vi "main.vi"() -> ()   [LabVIEW 2026]
uses:
  controls/message.ctl
  controls/data.ctl
  controls/channels.ctl
  controls/init cluster.ctl
  <instrlib>/Agilent 2000 3000 X-Series/Agilent 2000 3000 X-Series.lvlib
panel:
  out "times array":timestamp[](array[timestamp])
  in  "File Path":path
  out "results array 2":cluster{"V":dbl, "dV":dbl, "Q":dbl, "dQ":dbl}[](array[cluster])
  out "results array 1":cluster{"V":dbl, "dV":dbl, "Q":dbl, "dQ":dbl}[](array[cluster])
  in  "stop":bool
  out "dQ2":dbl
  out "Q2":dbl
  out "dV2":dbl
  out "V2":dbl
  out "dQ1":dbl
  out "Q1":dbl
  out "dV1":dbl
  out "V1":dbl
  in  "measure way":enum16{"single", "continuous"}(ring)
  in  "Testing":bool
  in  "Scope name":refnum<visa-resource-name>
  out "Initialized":bool
  in  "save":bool
  in  "Stop":bool
  in  "begin":bool
  out "Status":string
  in  "Tab Control":enum32{"Measurement Mode", "Tuning Mode"}(tab)
  out "output 2":waveform(dbl)(graph)
  out "output 1":waveform(dbl)(graph)
  in  "output 2 channel":T1(ring)
  in  "output 1 channel":T2(ring)
  out "output view":waveform(dbl)(graph)
  out "signal and timing":waveform(dbl)[](graph)
  # "CONTROLS"
  # "RESULTS - BCM 1"
  # "RESULTS - BCM 2"
  # "OPERATIONS"
  # "±"
  # "±"
  # "±"
  # "±"
  # "Save to location:"
  # "OUTPUT - BCM 1"
  # "OUTPUT - BCM 2"
  # "SIGNAL AND TIMING"
  # "OUTPUT"
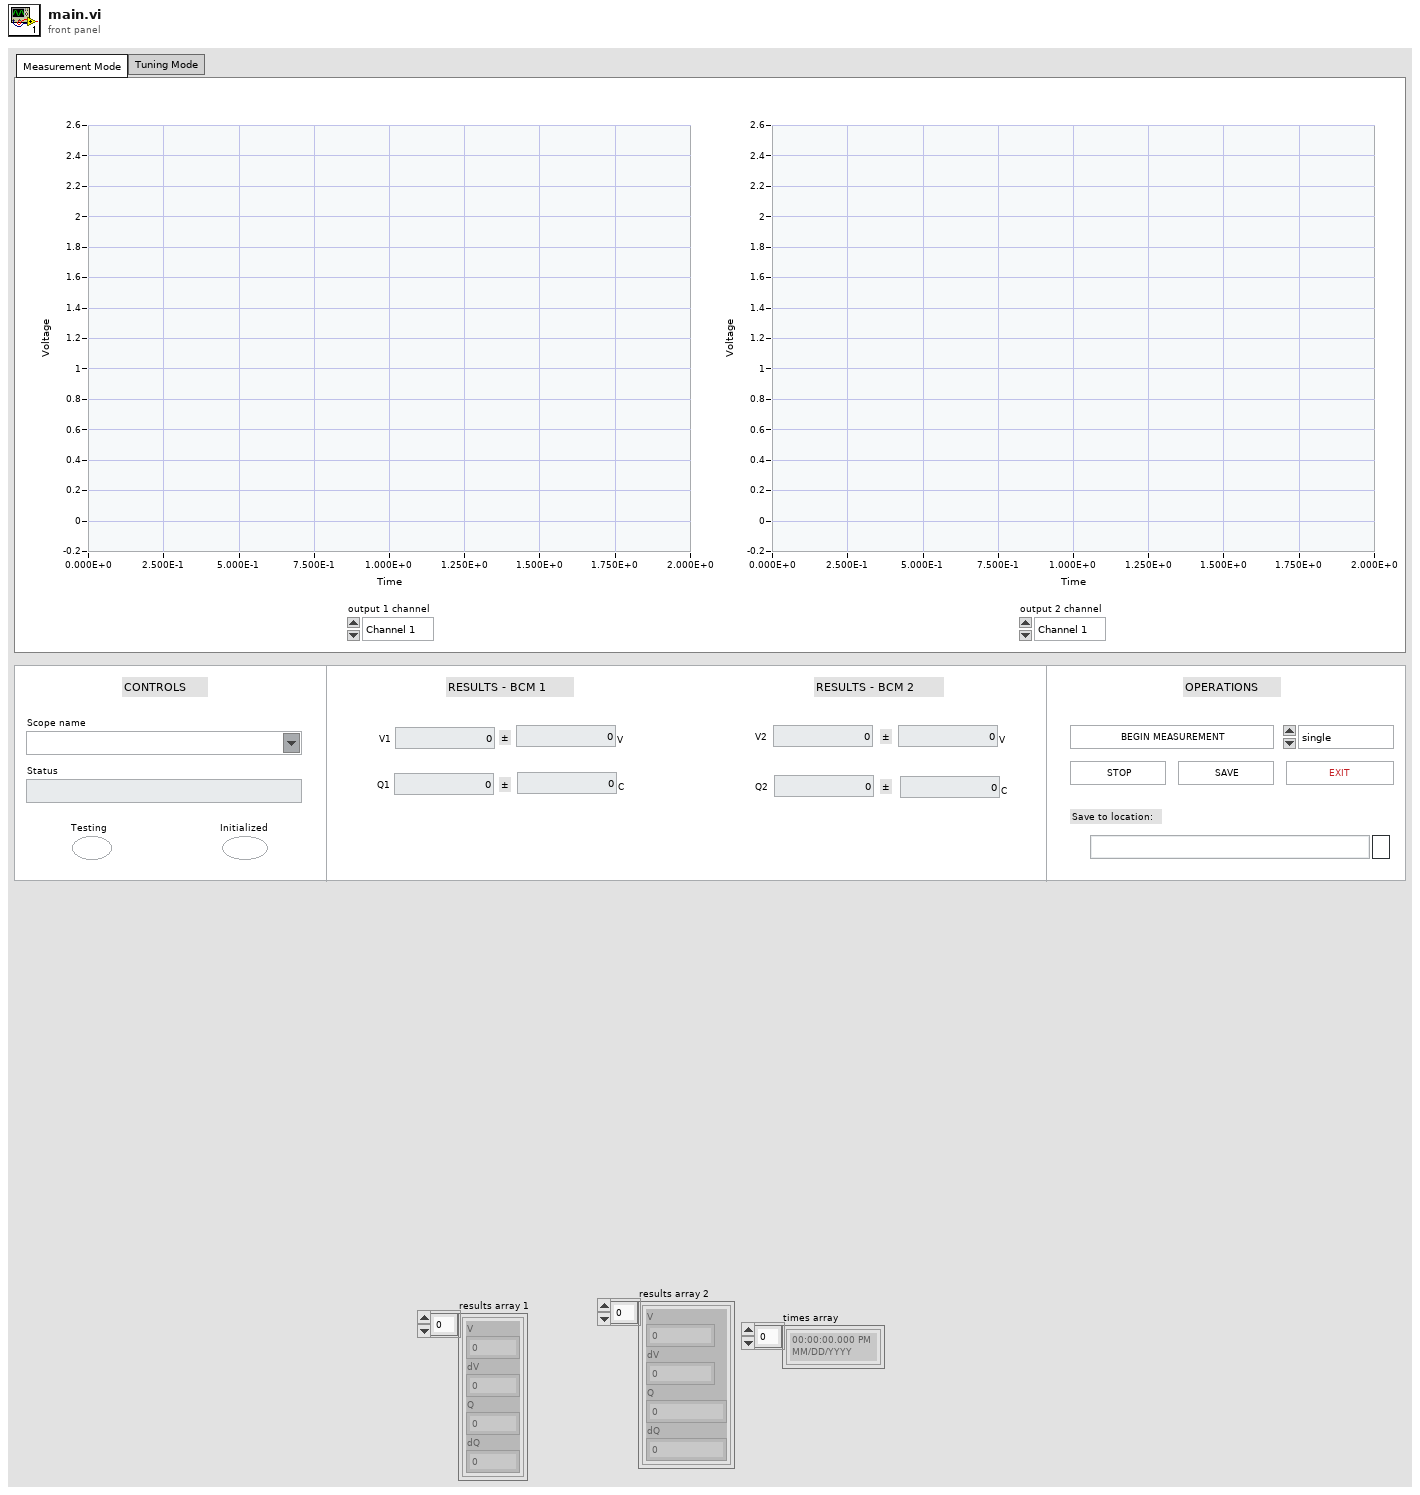
[diagram p1: front panel]
types:
  T1 = enum16{"Channel 1", "Channel 2", "Channel 3", "Channel 4"}
  T2 = enum32{"Channel 1", "Channel 2", "Channel 3", "Channel 4"}
  T3 = typedef "data.ctl" = cluster{"VISA resource name":refnum<visa-resource-name>, "error in":errorcluster}
  T4 = typedef "message.ctl" = cluster{"name":string, "Variant":variant}
  T5 = cluster{"results array 1":cluster{"V":dbl, "dV":dbl, "Q":dbl, "dQ":dbl}[], "results array 2":cluster{"V":dbl, "dV":dbl, "Q":dbl, "dQ":dbl}[], "times array":timestamp[]}
  T6 = typedef "init cluster.ctl" = cluster{"enable 1":bool, "enable 2":bool, "enable 3":bool, "enable 4":bool, "range 1":dbl, "range 2":dbl, "range 3":dbl, "range 4":dbl, "scale 1":dbl, "scale 2":dbl, "scale 3":dbl, "scale 4":dbl}
  T7 = enum8{"Enabled", "Disabled", "Disabled and Grayed Out"}
  T8 = typedef "channels.ctl" = i32
  T9 = enum32{"Channel 1", "Channel 2", "Channel 3", "Channel 4"}[]
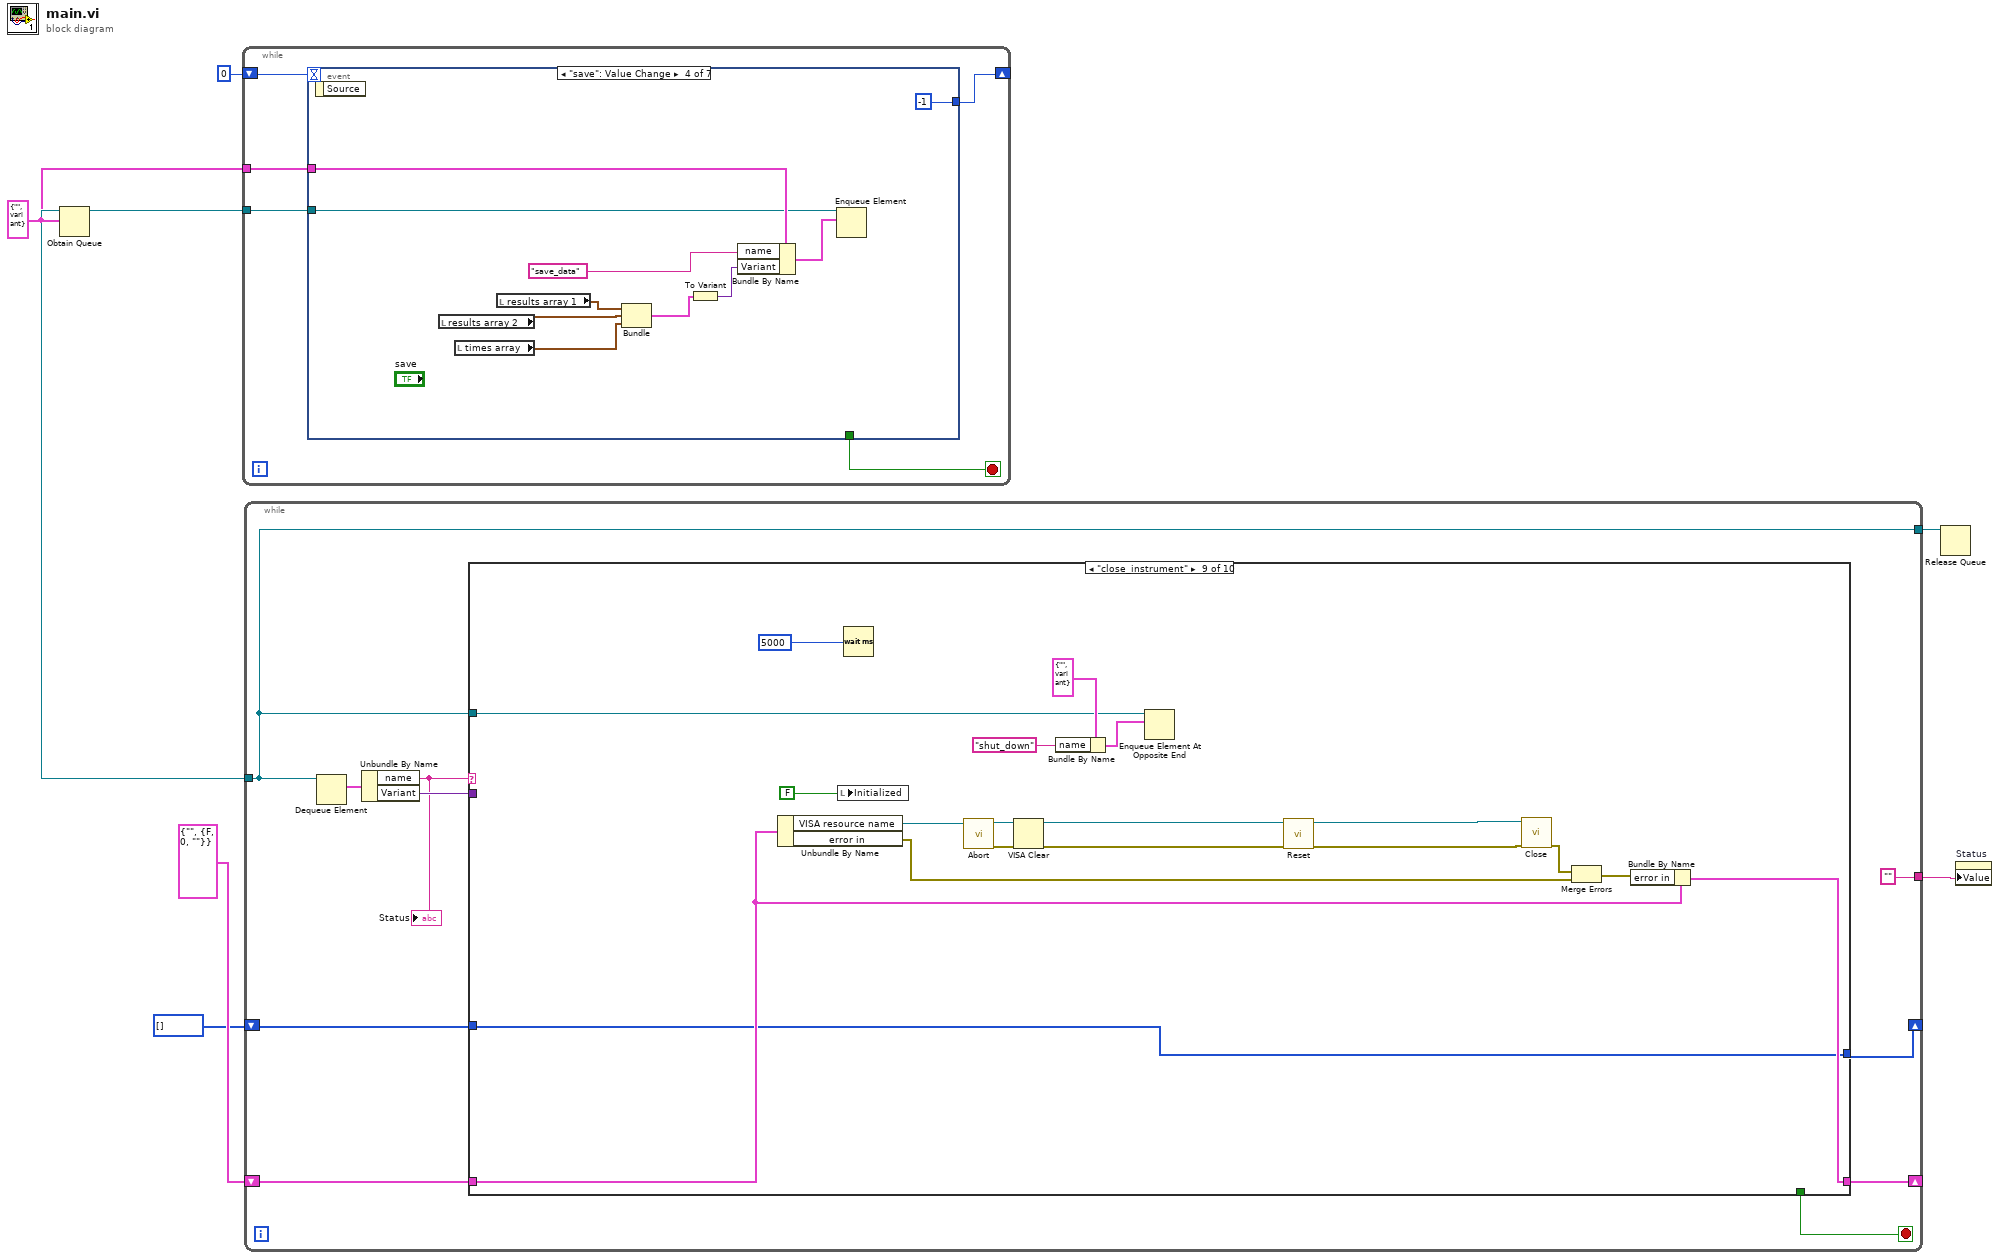
[diagram p0: block diagram]
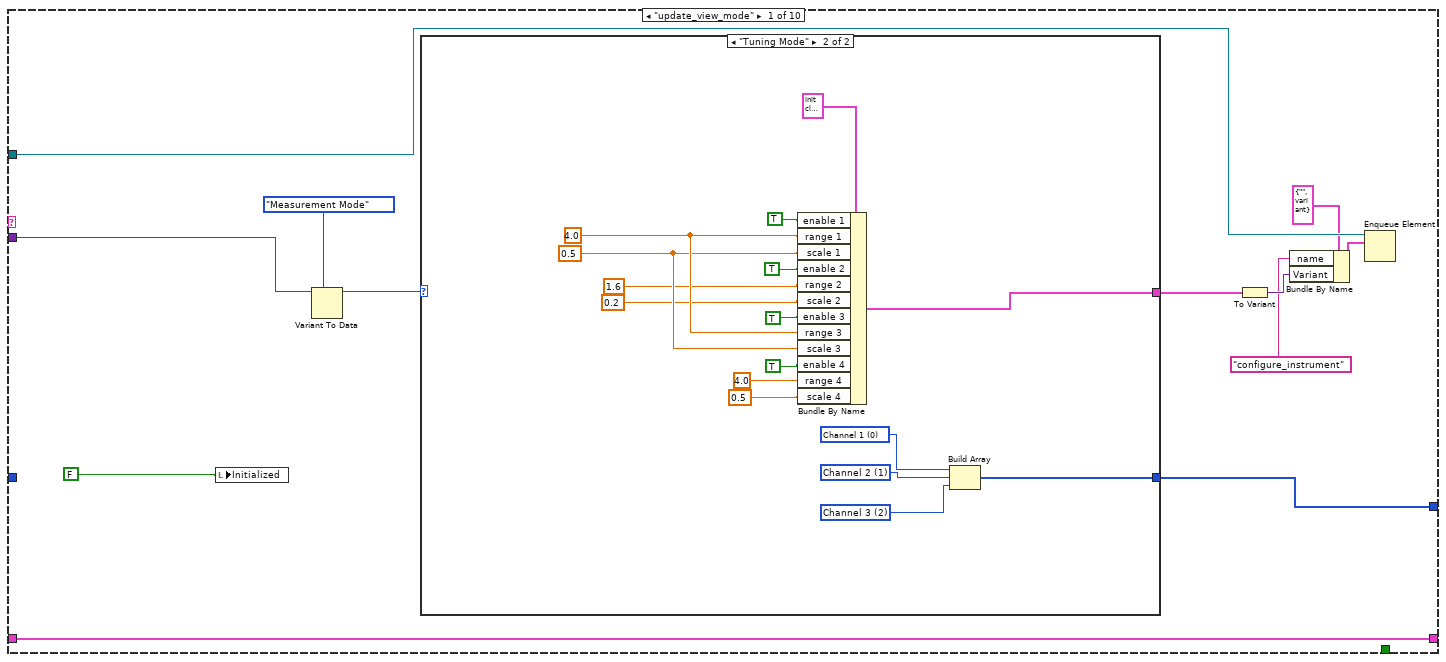
[diagram p2: hidden frame]
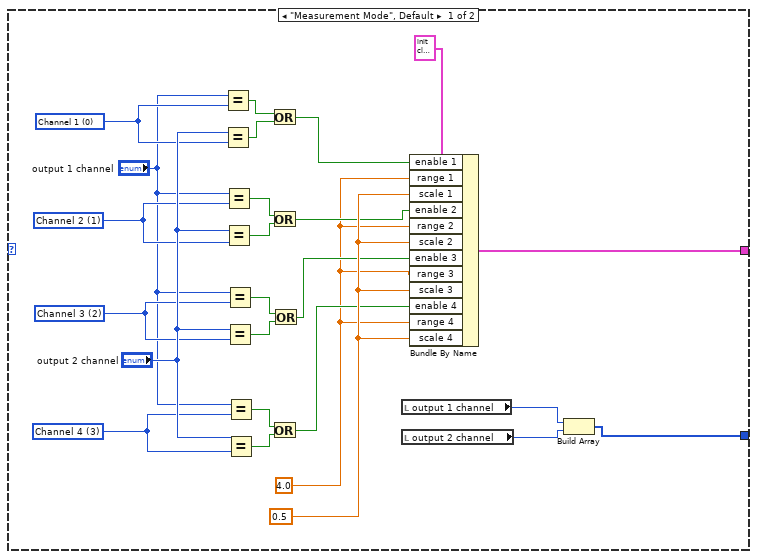
[diagram p3: hidden frame]
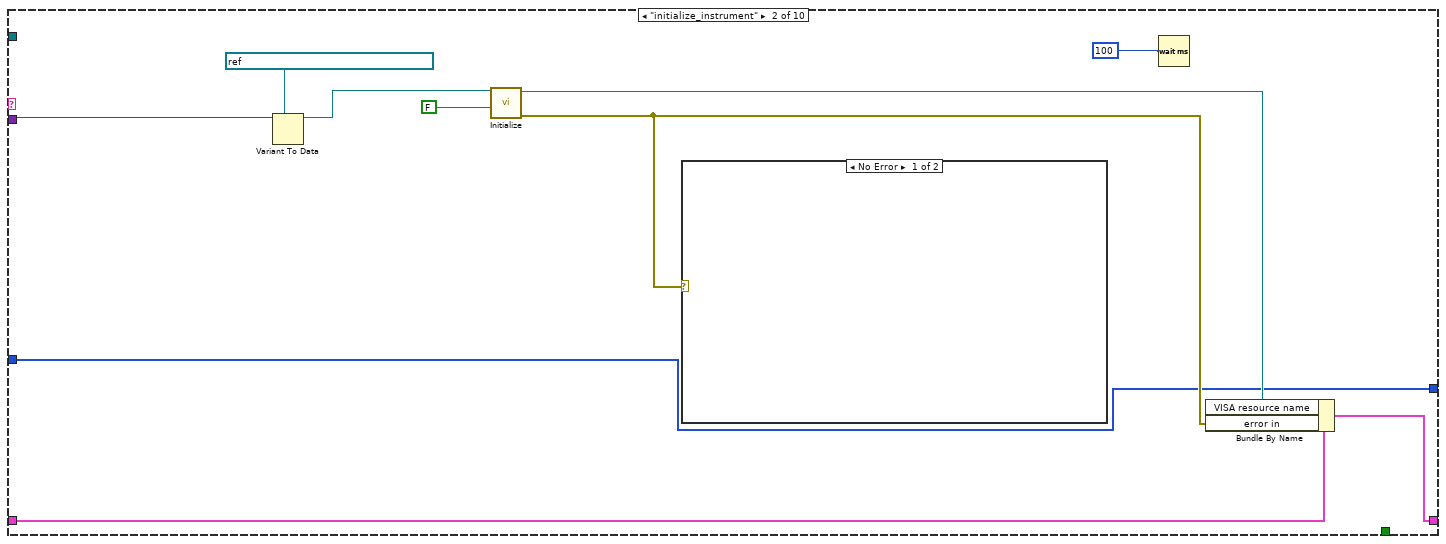
[diagram p4: hidden frame]
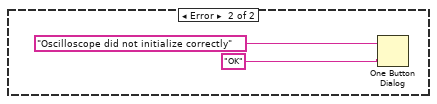
[diagram p5: hidden frame]
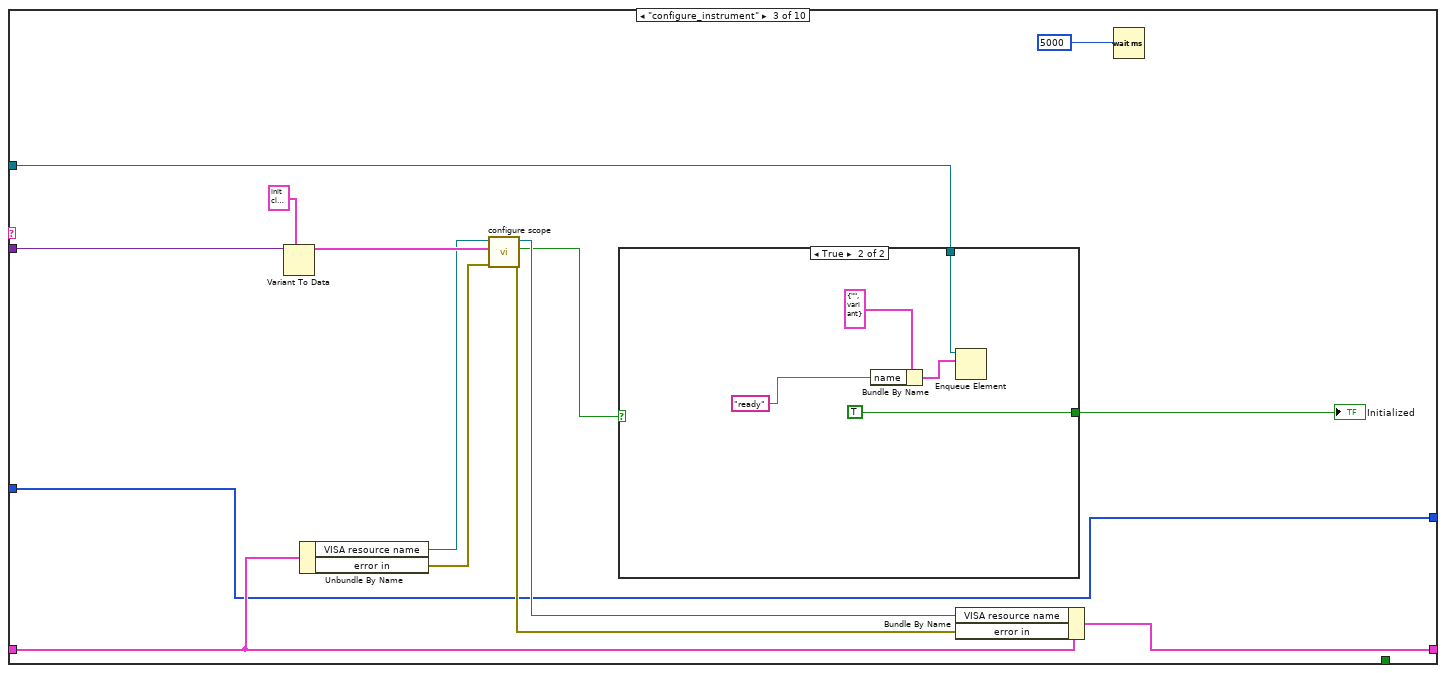
[diagram p6: hidden frame]
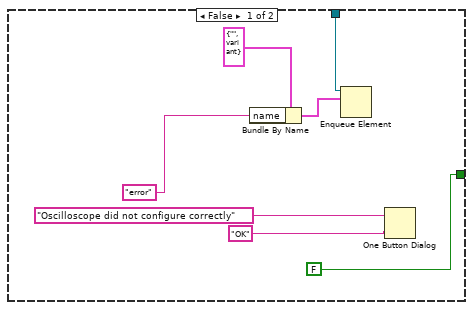
[diagram p7: hidden frame]
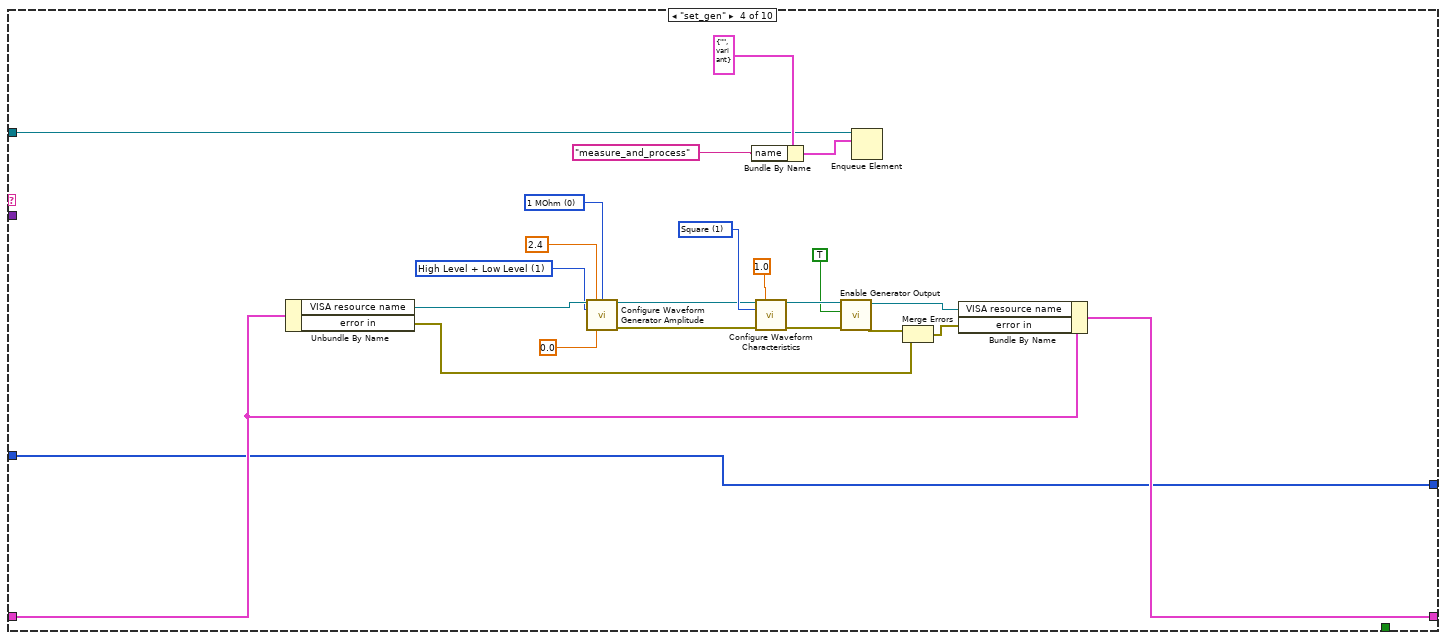
[diagram p8: hidden frame]
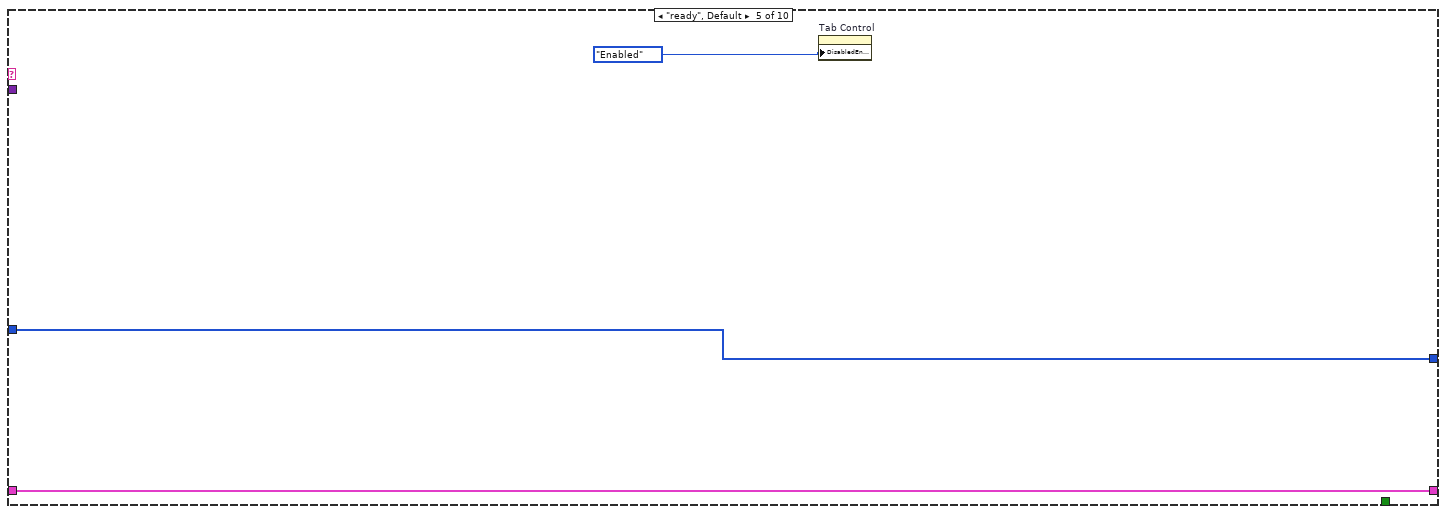
[diagram p9: hidden frame]
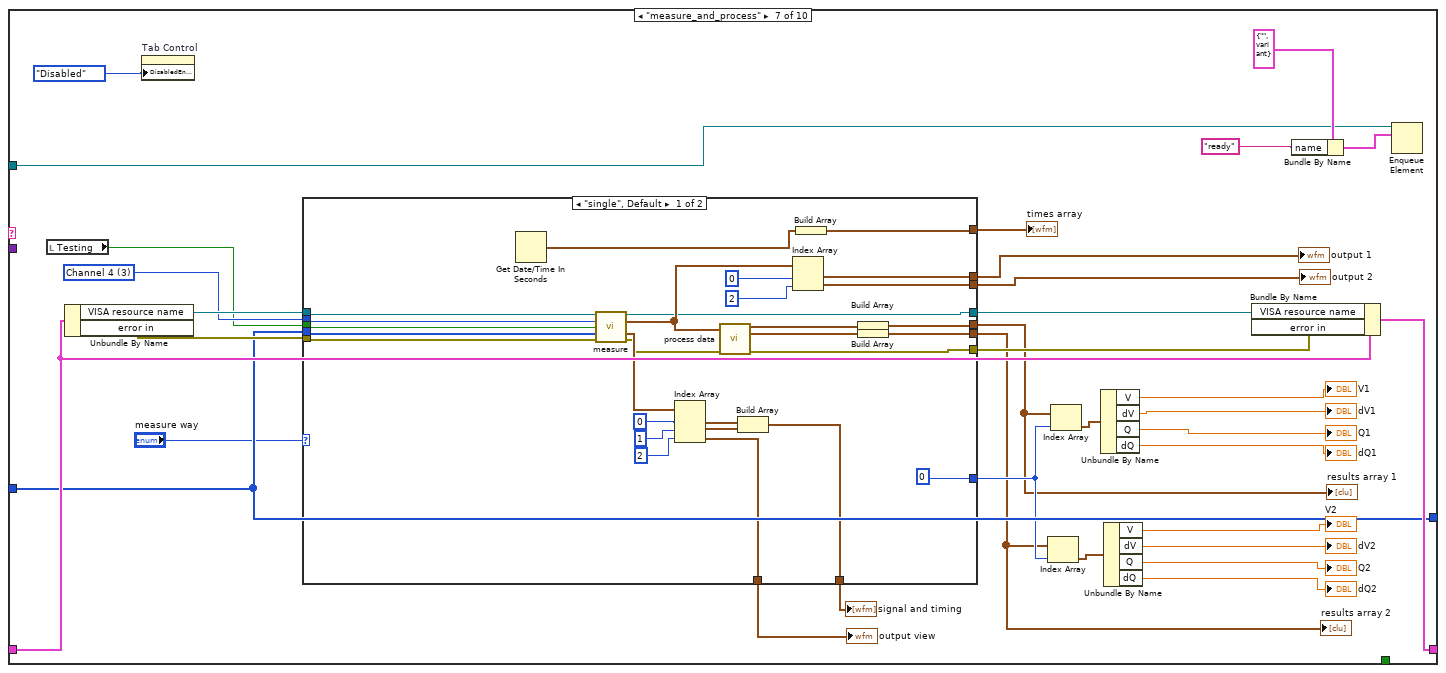
[diagram p11: hidden frame]
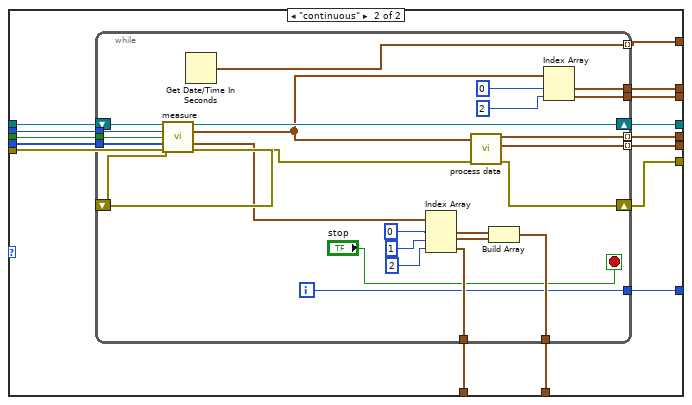
[diagram p12: hidden frame]
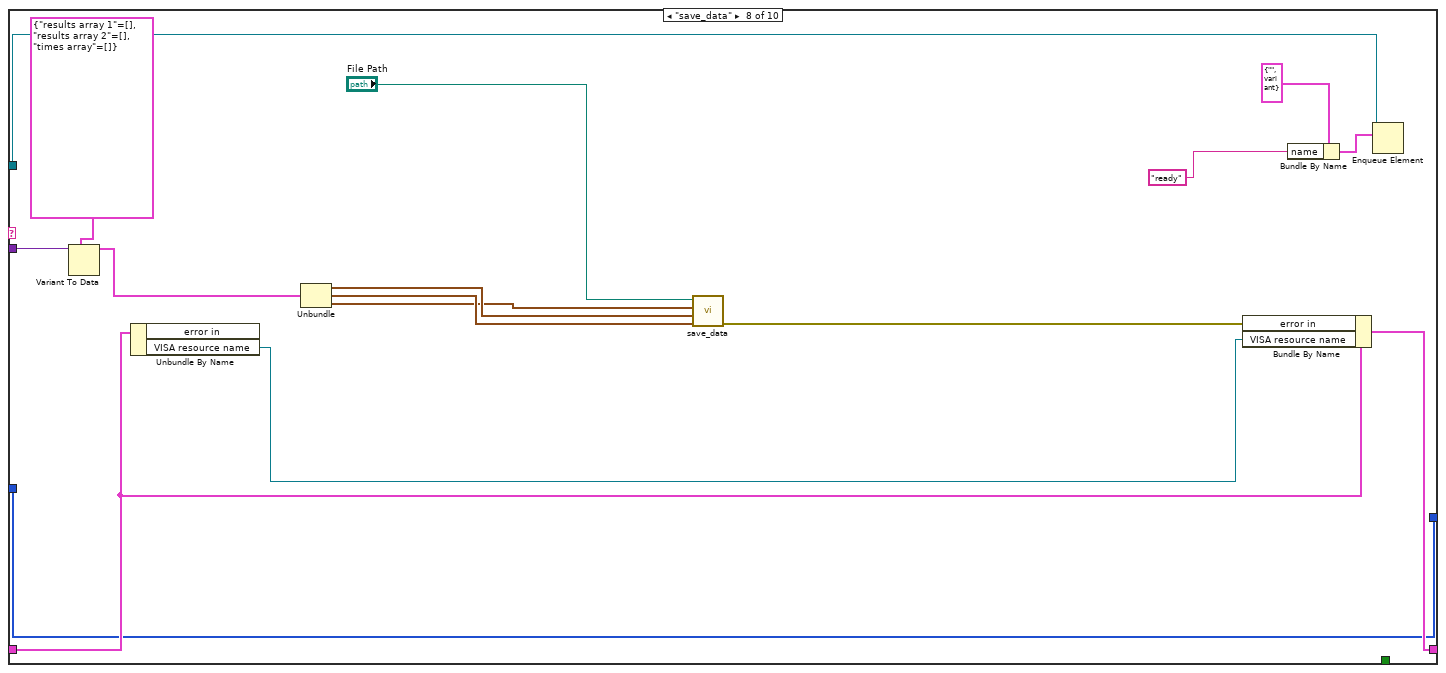
[diagram p13: hidden frame]
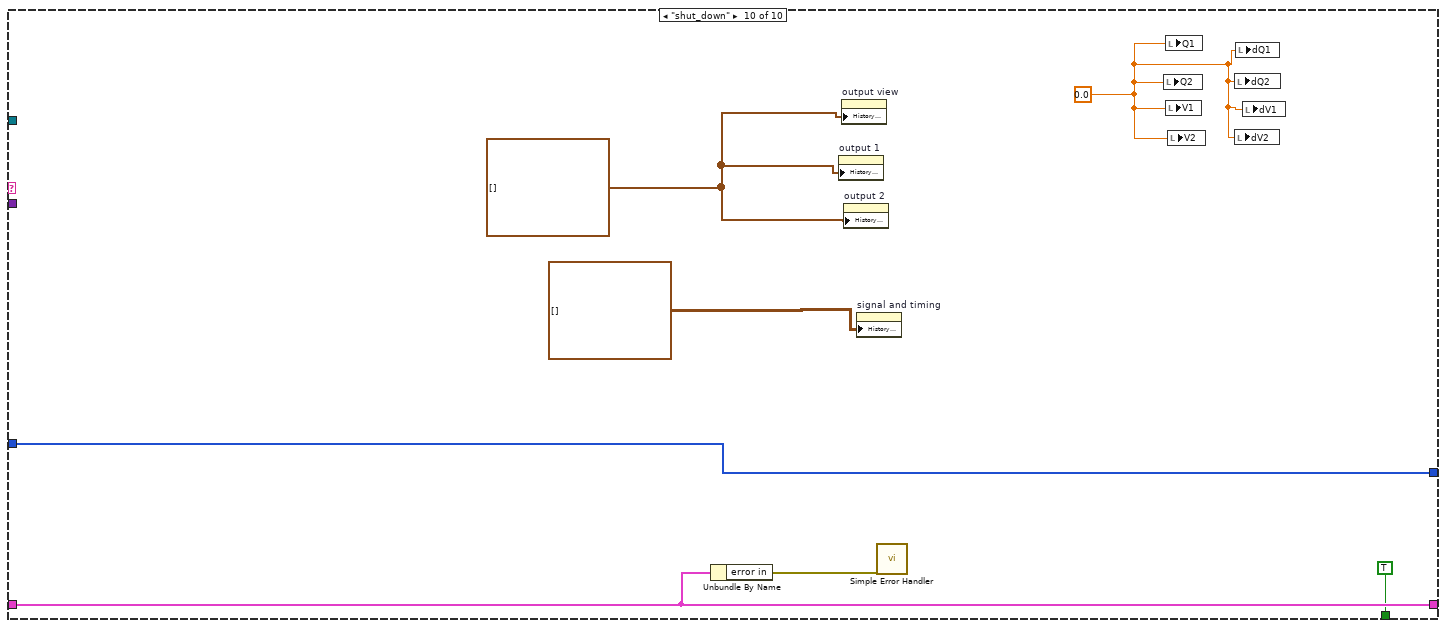
[diagram p14: hidden frame]
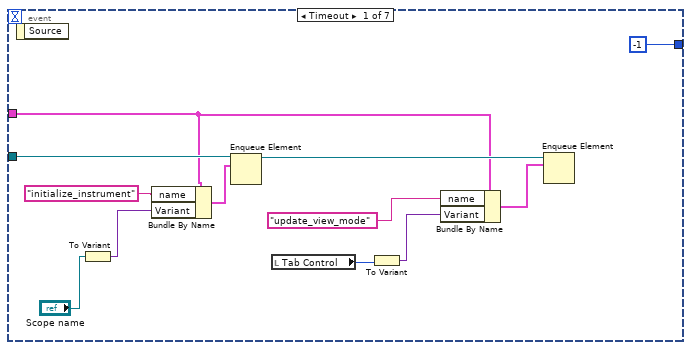
[diagram p15: hidden frame]
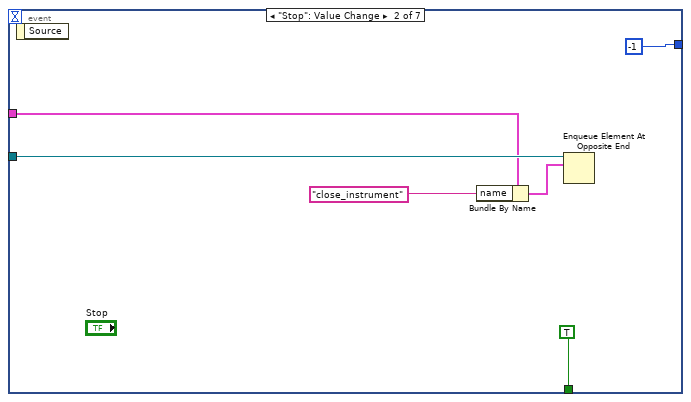
[diagram p16: hidden frame]
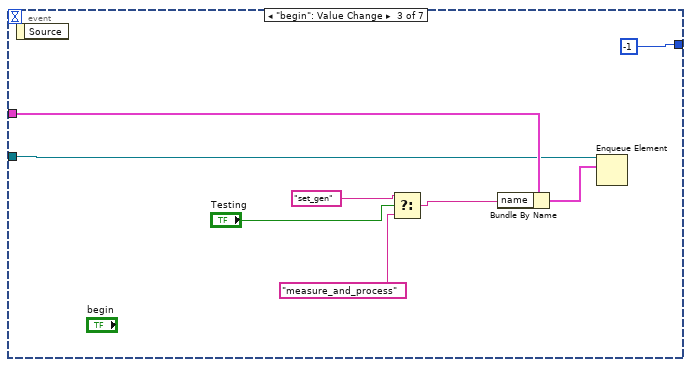
[diagram p17: hidden frame]
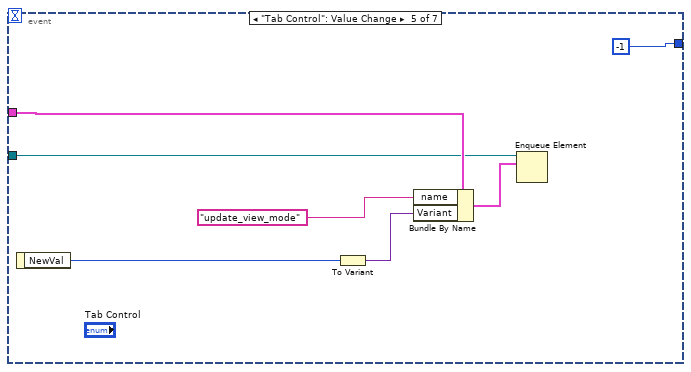
[diagram p18: hidden frame]
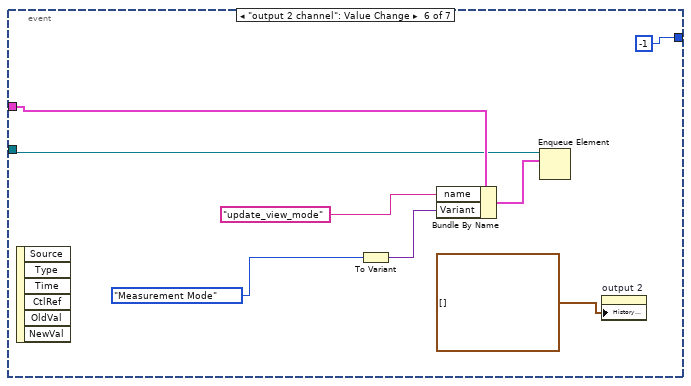
[diagram p19: hidden frame]
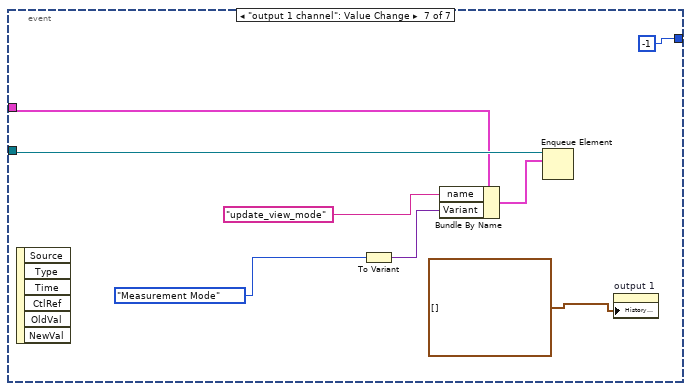
[diagram p20: hidden frame]
diagram:
  w4 = T4 {"name"="", "Variant"=variant} ("message")
  n1 = Obtain Queue(element data type=w4) -> (queue out=w6:refnum<queue>)  [unwired: 4 in, 2 out]
  n2 = while {
    shift-right: [w11] -> _
    shift-left: 0 -> [w12]
    tunnel: w6 -> [w8]
    tunnel: w4 -> [w9]
    stop <- w10 stop-if-true
    n3 = event shown="[3] \"save\": Value Change" {
      selector: _ -> [_ _ _ _ _ _ _]
      dyn-events: _ -> [_ _ _ _ _ _ _]
      timeout: w12 -> [_ _ _ _ _ _ _]
      tunnel: [-1 -1 -1 -1 -1 -1 -1] -> w11
      tunnel: [_ TRUE _ _ _ _ _] -> w10
      tunnel: w9 -> [w15 w28 w37 w46 w53 w59 w65]
      tunnel: w8 -> [w19 w29 w36 w45 w52 w58 w66]
      event Timeout {
        n4 = event-data() -> ()  [unwired: 1 in, 1 out]
        n5 = To Variant(anything="Scope name") -> (Variant=w17:variant)
        n6 = Bundle By Name(cluster=w15, "name"="initialize_instrument", "Variant"=w17) -> (w16:T4)
        n7 = Enqueue Element(queue=w19, element=w16) -> (queue out=w18:refnum<queue>)  [unwired: 2 in, 2 out]
        n8 = local read "Tab Control"() -> (w20:enum32{"Measurement Mode", "Tuning Mode"})
        n9 = To Variant(anything=w20) -> (Variant=w23:variant)
        n10 = Bundle By Name(cluster=w15, "name"="update_view_mode", "Variant"=w23) -> (w21:T4)
        n11 = Enqueue Element(queue=w18, element=w21) -> ()  [unwired: 2 in, 3 out]
      }
      event "Stop": Value Change {
        n12 = event-data() -> ()  [unwired: 1 in, 1 out]
        n13 = Bundle By Name(cluster=w28, "name"="close_instrument") -> (w27:T4)
        n14 = Enqueue Element At Opposite End(queue=w29, element=w27) -> ()  [unwired: 2 in, 3 out]
      }
      event "begin": Value Change {
        n15 = event-data() -> ()  [unwired: 1 in, 1 out]
        n16 = Select(t="set_gen", s="Testing", f="measure_and_process") -> (s? t:f=w31:string)
        n17 = Bundle By Name(cluster=w37, "name"=w31) -> (w38:T4)
        n18 = Enqueue Element(queue=w36, element=w38) -> ()  [unwired: 2 in, 3 out]
      }
      event "save": Value Change {
        n19 = event-data() -> ()  [unwired: 1 in, 1 out]
        n20 = local read "results array 2"() -> (w42:cluster{"V":dbl, "dV":dbl, "Q":dbl, "dQ":dbl}[])
        n21 = local read "times array"() -> (w39:timestamp[])
        n22 = local read "results array 1"() -> (w43:cluster{"V":dbl, "dV":dbl, "Q":dbl, "dQ":dbl}[])
        n23 = Bundle("results array 1"=w43, "results array 2"=w42, "times array"=w39) -> (w40:T5)  [unwired: 1 in]
        n24 = To Variant(anything=w40) -> (Variant=w41:variant)
        n25 = Bundle By Name(cluster=w46, "name"="save_data", "Variant"=w41) -> (w47:T4)
        n26 = Enqueue Element(queue=w45, element=w47) -> ()  [unwired: 2 in, 3 out]
      }
      event "Tab Control": Value Change {
        n27 = event-data() -> ("NewVal"=w51:enum32{"Measurement Mode", "Tuning Mode"})  [unwired: 1 in]
        n28 = To Variant(anything=w51) -> (Variant=w50:variant)
        n29 = Bundle By Name(cluster=w53, "name"="update_view_mode", "Variant"=w50) -> (w54:T4)
        n30 = Enqueue Element(queue=w52, element=w54) -> ()  [unwired: 2 in, 3 out]
      }
      event "output 2 channel": Value Change {
        n31 = event-data() -> ()  [unwired: 1 in, 6 out]
        n32 = To Variant(anything=enum32{"Measurement Mode", "Tuning Mode"}."Measurement Mode" ("Tab Control")) -> (Variant=w63:variant)
        n33 = Bundle By Name(cluster=w59, "name"="update_view_mode", "Variant"=w63) -> (w62:T4)
        n34 = Enqueue Element(queue=w58, element=w62) -> ()  [unwired: 2 in, 3 out]
        n35 = property on="output 2" class="WFChart (strict)"("History Data"=waveform(dbl)[] []) -> ()  [unwired: 2 in, 2 out]
      }
      event "output 1 channel": Value Change {
        n36 = event-data() -> ()  [unwired: 1 in, 6 out]
        n37 = To Variant(anything=enum32{"Measurement Mode", "Tuning Mode"}."Measurement Mode" ("Tab Control")) -> (Variant=w70:variant)
        n38 = Bundle By Name(cluster=w65, "name"="update_view_mode", "Variant"=w70) -> (w71:T4)
        n39 = Enqueue Element(queue=w66, element=w71) -> ()  [unwired: 2 in, 3 out]
        n40 = property on="output 1" class="WFChart (strict)"("History Data"=waveform(dbl)[] []) -> ()  [unwired: 2 in, 2 out]
      }
    }
  }
  n41 = while {
    tunnel: w6 -> [w80]
    tunnel: [w80] -> w3
    shift-right: [w77] -> _
    shift-left: T3 {"VISA resource name"="", "error in"={"status"=FALSE, "code"=0, "source"=""}} ("data") -> [w78]
    shift-right: [w75] -> _
    shift-left: i32[] [] -> [w74]
    tunnel: [""] -> w1
    stop <- w76 stop-if-true
    n42 = Dequeue Element(queue=w80) -> (element=w81:T4)  [unwired: 2 in, 3 out]
    n43 = Unbundle By Name(w81) -> ("name"=w73:string, "Variant"=w79:variant)
    "Status" <- w73
    n44 = case shown="\"close_instrument\"" w73 {
      tunnel: w80 -> [w89 _ w147 w178 _ _ w229 w311 w329 _]
      tunnel: w79 -> [w93 w144 w159 _ _ _ _ w310 _ _]
      tunnel: w78 -> [w84 w141 w155 w180 w198 w200 w230 w317 w328 w343]
      tunnel: [w84 w139 w150 w179 w198 w200 w228 w316 w327 w343] -> w77
      tunnel: [_ _ _ _ _ _ _ _ _ TRUE] -> w76
      tunnel: [w83 w136 w148 w177 w197 w199 w222 w315 w323 w340] -> w75
      tunnel: w74 -> [_ w136 w148 w177 w197 w199 w222 w315 w323 w340]
      frame "update_view_mode" {
        n45 = local write "Initialized"(FALSE ("Initialized")) -> ()
        n46 = Variant To Data(type=enum32{"Measurement Mode", "Tuning Mode"}."Measurement Mode" ("Tab Control"), Variant=w93) -> (data=w91:enum32{"Measurement Mode", "Tuning Mode"})  [unwired: 1 in, 1 out]
        n47 = case shown="\"Tuning Mode\"" w91 {
          tunnel: [w97 w125] -> w90
          tunnel: [w94 w124] -> w83
          frame "Measurement Mode", Default {
            w98 = 4.0
            w103 = 0.5
            w114 = T8 3 items=["Channel 1", "Channel 2", "Channel 3", "Channel 4"] ("Channel Name (0: Channel 1)")
            w115 = T8 2 items=["Channel 1", "Channel 2", "Channel 3", "Channel 4"] ("Channel Name (0: Channel 1)")
            w116 = T8 1 items=["Channel 1", "Channel 2", "Channel 3", "Channel 4"] ("Channel Name (0: Channel 1)")
            w117 = T8 0 items=["Channel 1", "Channel 2", "Channel 3", "Channel 4"] ("Channel Name (0: Channel 1)")
            n48 = Equal?(x="output 1 channel", y=w117) -> (x = y?=w112:bool)
            n49 = Equal?(x="output 2 channel", y=w117) -> (x = y?=w111:bool)
            n50 = Equal?(x="output 1 channel", y=w116) -> (x = y?=w110:bool)
            n51 = Equal?(x="output 2 channel", y=w116) -> (x = y?=w109:bool)
            n52 = Equal?(x="output 1 channel", y=w115) -> (x = y?=w108:bool)
            n53 = Equal?(x="output 2 channel", y=w115) -> (x = y?=w107:bool)
            n54 = Equal?(x="output 1 channel", y=w114) -> (x = y?=w106:bool)
            n55 = Equal?(x="output 2 channel", y=w114) -> (x = y?=w105:bool)
            n56 = Or(x=w112, y=w111) -> (x .or. y?=w99:bool)
            n57 = Or(x=w110, y=w109) -> (x .or. y?=w100:bool)
            n58 = Or(x=w106, y=w105) -> (x .or. y?=w102:bool)
            n59 = Or(x=w108, y=w107) -> (x .or. y?=w101:bool)
            n60 = local read "output 1 channel"() -> (w96:T2)
            n61 = local read "output 2 channel"() -> (w95:T1)
            n62 = Bundle By Name(cluster=T6 {"enable 1"=FALSE, "enable 2"=FALSE, "enable 3"=FALSE, "enable 4"=FALSE, "range 1"=0.0, "range 2"=0.0, "range 3"=0.0, "range 4"=0.0, "scale 1"=0.0, "scale 2"=0.0, "scale 3"=0.0, "scale 4"=0.0} ("Init cluster"), "enable 1"=w99, "range 1"=w98, "scale 1"=w103, "enable 2"=w100, "range 2"=w98, "scale 2"=w103, "enable 3"=w101, "range 3"=w98, "scale 3"=w103, "enable 4"=w102, "range 4"=w98, "scale 4"=w103) -> (w97:T6)
            n63 = Build Array(w96, w95) -> (w94:T9)
          }
          frame "Tuning Mode" {
            w121 = 2 items=["Channel 1", "Channel 2", "Channel 3", "Channel 4", "External"] ("Trigger Level Source (0: Channel 1)")
            w122 = 1 items=["Channel 1", "Channel 2", "Channel 3", "Channel 4", "External"] ("Trigger Level Source (0: Channel 1)")
            w123 = 0 items=["Channel 1", "Channel 2", "Channel 3", "Channel 4", "External"] ("Trigger Level Source (0: Channel 1)")
            w128 = 0.5 ("scale 1")
            w129 = 4.0 ("range 1")
            n64 = Bundle By Name(cluster=T6 {"enable 1"=FALSE, "enable 2"=FALSE, "enable 3"=FALSE, "enable 4"=FALSE, "range 1"=0.0, "range 2"=0.0, "range 3"=0.0, "range 4"=0.0, "scale 1"=0.0, "scale 2"=0.0, "scale 3"=0.0, "scale 4"=0.0} ("Init cluster"), "enable 1"=TRUE, "range 1"=w129, "scale 1"=w128, "enable 2"=TRUE, "range 2"=1.6, "scale 2"=0.2, "enable 3"=TRUE, "range 3"=w129, "scale 3"=w128, "enable 4"=TRUE, "range 4"=4.0 ("range 1"), "scale 4"=0.5) -> (w125:T6)
            n65 = Build Array(w123, w122, w121) -> (w124:i32[])
          }
        }
        n66 = To Variant(anything=w90) -> (Variant=w86:variant)
        n67 = Bundle By Name(cluster=T4 {"name"="", "Variant"=variant} ("element"), "name"="configure_instrument", "Variant"=w86) -> (w88:T4)
        n68 = Enqueue Element(queue=w89, element=w88) -> ()  [unwired: 2 in, 3 out]
      }
      frame "initialize_instrument" {
        n69 = Variant To Data(type=refnum<visa-resource-name> "TCPIP0::192.168.1.11::inst0::INSTR" ("Device name"), Variant=w144) -> (data=w137:refnum<visa-resource-name>)  [unwired: 1 in, 1 out]
        n70 = call <instrlib>:"Initialize.vi"("Reset (True)"=FALSE, "VISA resource name"=w137) -> ("error out"=w138:errorcluster, "VISA resource name out"=w140:refnum<visa-resource-name>)  [unwired: 8 in]
        n71 = case shown="No Error" w138 {
          frame No Error {
          }
          frame Error {
            n72 = One Button Dialog(message="Oscilloscope did not initialize correctly", button name ("OK")="OK") -> ()  [unwired: 1 out]
          }
        }
        n73 = Wait (ms)(milliseconds to wait=u32 100) -> ()  [unwired: 1 out]
        n74 = Bundle By Name(cluster=w141, "VISA resource name"=w140, "error in"=w138) -> (w139:T3)
      }
      frame "configure_instrument" {
        n75 = Variant To Data(type=T6 {"enable 1"=FALSE, "enable 2"=FALSE, "enable 3"=FALSE, "enable 4"=FALSE, "range 1"=0.0, "range 2"=0.0, "range 3"=0.0, "range 4"=0.0, "scale 1"=0.0, "scale 2"=0.0, "scale 3"=0.0, "scale 4"=0.0} ("Init cluster"), Variant=w159) -> (data=w158:T6)  [unwired: 1 in, 1 out]
        n76 = Unbundle By Name(w155) -> ("VISA resource name"=w156:refnum<visa-resource-name>, "error in"=w157:errorcluster)
        n77 = call "configure scope.vi"("error in"=w157, "Init cluster"=w158, "VISA resource name I"=w156) -> ("error out"=w153:errorcluster, "ready"=w152:bool, "VISA resource name O"=w154:refnum<visa-resource-name>)  [unwired: 6 in]
        n78 = case shown="True" w152 {
          tunnel: [FALSE ("Initialized") TRUE ("Initialized")] -> w149
          tunnel: w147 -> [w161 w168]
          frame False {
            n79 = Bundle By Name(cluster=T4 {"name"="", "Variant"=variant} ("message"), "name"="error" ("f")) -> (w164:T4)
            n80 = Enqueue Element(queue=w161, element=w164) -> ()  [unwired: 2 in, 3 out]
            n81 = One Button Dialog(message="Oscilloscope did not configure correctly", button name ("OK")="OK") -> ()  [unwired: 1 out]
          }
          frame True {
            n82 = Bundle By Name(cluster=T4 {"name"="", "Variant"=variant} ("message"), "name"="ready" ("f")) -> (w171:T4)
            n83 = Enqueue Element(queue=w168, element=w171) -> ()  [unwired: 2 in, 3 out]
          }
        }
        "Initialized" <- w149
        n84 = Bundle By Name(cluster=w155, "VISA resource name"=w154, "error in"=w153) -> (w150:T3)
        n85 = Wait (ms)(milliseconds to wait=u32 5000) -> ()  [unwired: 1 out]
      }
      frame "set_gen" {
        w181 = 0 items=["1 MOhm", "50 Ohm"] ("Load Impedance (0: 1 MOhm)")
        w191 = 1 items=["Sine", "Square", "Ramp", "Pulse", "Noise", "DC", "Sine Cardinal", "Exponential Rise", "Exponential Fall", "Cardiac", "Gaussian Pulse", "Arbitrary"] ("Function Type (0: Sine)")
        w192 = 1 items=["Amplitude + Offset", "High Level + Low Level"] ("Setting Style (0: Amplitude + Offset)")
        n86 = Unbundle By Name(w180) -> ("VISA resource name"=w195:refnum<visa-resource-name>, "error in"=w173:errorcluster)
        n87 = call <instrlib>:"Configure Waveform Generator Amplitude.vi"("VISA resource name"=w195, "High Level (1.0 V)"=2.4, "Load Impedance (0: 1 MOhm)"=w181, "Setting Style (0: Amplitude + Offset)"=w192, "Low Level (0.0 V)"=0.0) -> ("VISA resource name out"=w190:refnum<visa-resource-name>, "error out"=w189:errorcluster)  [unwired: 9 in]
        n88 = Bundle By Name(cluster=T4 {"name"="", "Variant"=variant} ("message"), "name"="measure_and_process") -> (w183:T4)
        n89 = call <instrlib>:"Configure Waveform Characteristics.vi"("VISA resource name"=w190, "Period (0.001)"=1.0, "Function Type (0: Sine)"=w191, "error in (no error)"=w189) -> ("VISA resource name out"=w187:refnum<visa-resource-name>, "error out"=w188:errorcluster)  [unwired: 10 in]
        n90 = call <instrlib>:"Enable Generator Output.vi"("error in (no error)"=w188, "Enable Output (F: Disable)"=TRUE, "VISA resource name"=w187) -> ("error out"=w175:errorcluster, "VISA resource name out"=w185:refnum<visa-resource-name>)  [unwired: 7 in]
        n91 = Enqueue Element(queue=w178, element=w183) -> ()  [unwired: 2 in, 3 out]
        n92 = Merge Errors(w175, w173) -> (w174:errorcluster)
        n93 = Bundle By Name(cluster=w180, "VISA resource name"=w185, "error in"=w174) -> (w179:T3)
      }
      frame "ready", Default {
        n94 = property on="Tab Control" class="TabCtl (strict)"("DisabledEnum"=T7."Enabled" ("Disabled")) -> ()  [unwired: 2 in, 2 out]
      }
      frame "error" {
      }
      frame "measure_and_process" {
        w224 = 3 items=["Channel 1", "Channel 2", "Channel 3", "Channel 4", "External"] ("Trigger Channel")
        n95 = local read "Testing"() -> (w223:bool)
        n96 = Unbundle By Name(w230) -> ("VISA resource name"=w226:refnum<visa-resource-name>, "error in"=w225:errorcluster)
        n97 = property on="Tab Control" class="TabCtl (strict)"("DisabledEnum"=T7."Disabled" ("Disabled")) -> ()  [unwired: 2 in, 2 out]
        n98 = case shown="\"single\", Default" "measure way" {
          tunnel: w226 -> [w247 w276]
          tunnel: w225 -> [w243 w275]
          tunnel: w224 -> [w246 w274]
          tunnel: w223 -> [w245 w273]
          tunnel: w222 -> [w244 w272]
          tunnel: [w251 w271] -> w221
          tunnel: [w250 w270] -> w220
          tunnel: [w249 w269] -> w219
          tunnel: [w248 w268] -> w218
          tunnel: [w239 w264] -> w203
          tunnel: [w237 w267] -> w202
          tunnel: [w242 w266] -> w208
          tunnel: [w241 w265] -> w207
          tunnel: [0 w263] -> w205
          tunnel: [w235 w262] -> w201
          frame "single", Default {
            n99 = Get Date/Time In Seconds() -> (seconds since 1Jan1904=w234:timestamp)
            n100 = call "measure.vi"("VISA resource name I"=w247, "Trigger Channel"=w246, "Testing?"=w245, "Channels"=w244, "error in"=w243) -> ("VISA resouce name O"=w251:refnum<visa-resource-name>, "measurement results"=w252:waveform(dbl)[], "Tuning results"=w259:waveform(dbl)[], "error out"=w253:errorcluster)  [unwired: 7 in]
            n101 = Index Array(array=w259, index #1=0 ("index"), index #2=1 ("index"), index #3=2 ("index")) -> (element #1=w255:waveform(dbl), element #2=w254:waveform(dbl), element #3=w241:waveform(dbl))
            n102 = call "process data.vi"("waveform array"=w252, "error in"=w253) -> ("device 1"=w240:cluster{"V":dbl, "dV":dbl, "Q":dbl, "dQ":dbl}, "device 2"=w238:cluster{"V":dbl, "dV":dbl, "Q":dbl, "dQ":dbl}, "error out"=w248:errorcluster)  [unwired: 11 in]
            n103 = Build Array(w255, w254) -> (w242:waveform(dbl)[])
            n104 = Index Array(array=w252, index #1=0 ("index"), index #2=2 ("index")) -> (element #1=w250:waveform(dbl), element #2=w249:waveform(dbl))
            n105 = Build Array(w234) -> (w235:timestamp[])
            n106 = Build Array(w240) -> (w239:cluster{"V":dbl, "dV":dbl, "Q":dbl, "dQ":dbl}[])
            n107 = Build Array(w238) -> (w237:cluster{"V":dbl, "dV":dbl, "Q":dbl, "dQ":dbl}[])
          }
          frame "continuous" {
            n108 = while {
              tunnel: w274 -> [w300]
              tunnel: w273 -> [w299]
              tunnel: w272 -> [w298]
              tunnel: [w294] -> w270
              tunnel: [w293] -> w269
              tunnel: [w283] -> w264 mode=indexing
              tunnel: [w282] -> w267 mode=indexing
              shift-right: [w297] -> w271
              shift-left: w276 -> [w302]
              shift-right: [w284] -> w268
              shift-left: w275 -> [w301]
              tunnel: [w281] -> w266
              tunnel: [w280] -> w265
              tunnel: [w278] -> w263
              tunnel: [w277] -> w262 mode=indexing
              i -> [w278]
              stop <- "stop" stop-if-true
              n109 = call "measure.vi"("VISA resource name I"=w302, "Trigger Channel"=w300, "Testing?"=w299, "Channels"=w298, "error in"=w301) -> ("VISA resouce name O"=w297:refnum<visa-resource-name>, "measurement results"=w285:waveform(dbl)[], "Tuning results"=w292:waveform(dbl)[], "error out"=w286:errorcluster)  [unwired: 7 in]
              n110 = Get Date/Time In Seconds() -> (seconds since 1Jan1904=w277:timestamp)
              n111 = Index Array(array=w292, index #1=0 ("index"), index #2=1 ("index"), index #3=2 ("index")) -> (element #1=w288:waveform(dbl), element #2=w287:waveform(dbl), element #3=w280:waveform(dbl))
              n112 = call "process data.vi"("waveform array"=w285, "error in"=w286) -> ("device 1"=w283:cluster{"V":dbl, "dV":dbl, "Q":dbl, "dQ":dbl}, "device 2"=w282:cluster{"V":dbl, "dV":dbl, "Q":dbl, "dQ":dbl}, "error out"=w284:errorcluster)  [unwired: 11 in]
              n113 = Build Array(w288, w287) -> (w281:waveform(dbl)[])
              n114 = Index Array(array=w285, index #1=0 ("index"), index #2=2 ("index")) -> (element #1=w294:waveform(dbl), element #2=w293:waveform(dbl))
            }
          }
        }
        "output 2" <- w219
        "output 1" <- w220
        "signal and timing" <- w208
        "output view" <- w207
        "results array 1" <- w203
        "results array 2" <- w202
        "times array" <- w201
        n115 = Index Array(array=w202, index=w205) -> (element=w204:cluster{"V":dbl, "dV":dbl, "Q":dbl, "dQ":dbl})
        n116 = Index Array(array=w203, index=w205) -> (element=w206:cluster{"V":dbl, "dV":dbl, "Q":dbl, "dQ":dbl})
        n117 = Unbundle By Name(w206) -> ("V"=→"V1":dbl, "dV"=→"dV1":dbl, "Q"=→"Q1":dbl, "dQ"=→"dQ1":dbl)
        n118 = Unbundle By Name(w204) -> ("V"=→"V2":dbl, "dV"=→"dV2":dbl, "Q"=→"Q2":dbl, "dQ"=→"dQ2":dbl)
        n119 = Bundle By Name(cluster=w230, "VISA resource name"=w221, "error in"=w218) -> (w228:T3)
        n120 = Bundle By Name(cluster=T4 {"name"="", "Variant"=variant} ("message"), "name"="ready") -> (w232:T4)
        n121 = Enqueue Element(queue=w229, element=w232) -> ()  [unwired: 2 in, 3 out]
      }
      frame "save_data" {
        n122 = Variant To Data(type=T5 {"results array 1"=[], "results array 2"=[], "times array"=[]} ("output cluster"), Variant=w310) -> (data=w309:T5)  [unwired: 1 in, 1 out]
        n123 = Unbundle By Name(w317) -> ("VISA resource name"=w318:refnum<visa-resource-name>)  [unwired: 1 out]
        n124 = Unbundle(w309) -> ("results array 1"=w308:cluster{"V":dbl, "dV":dbl, "Q":dbl, "dQ":dbl}[], "results array 2"=w307:cluster{"V":dbl, "dV":dbl, "Q":dbl, "dQ":dbl}[], "times array"=w303:timestamp[])
        n125 = call "save_data.vi"("data 2"=w307, "data 1"=w308, "times"=w303, "Filepath"="File Path") -> ("error out"=w306:errorcluster)  [unwired: 7 in]
        n126 = Bundle By Name(cluster=w317, "error in"=w306, "VISA resource name"=w318) -> (w316:T3)
        n127 = Bundle By Name(cluster=T4 {"name"="", "Variant"=variant} ("message"), "name"="ready" ("f")) -> (w313:T4)
        n128 = Enqueue Element(queue=w311, element=w313) -> ()  [unwired: 2 in, 3 out]
      }
      frame "close_instrument" {
        n129 = Unbundle By Name(w328) -> ("VISA resource name"=w337:refnum<visa-resource-name>, "error in"=w326:errorcluster)
        n130 = local write "Initialized"(FALSE ("ready?")) -> ()
        n131 = Wait (ms)(milliseconds to wait=u32 5000) -> ()  [unwired: 1 out]
        n132 = call <instrlib>:"Abort.vi"("VISA resource name"=w337) -> ("error out"=w330:errorcluster, "VISA resource name out"=w331:refnum<visa-resource-name>)  [unwired: 9 in]
        n133 = VISA Clear(VISA resource name=w331, error in (no error)=w330) -> (VISA resource name out=w321:refnum<visa-resource-name>, error out=w322:errorcluster)
        n134 = Bundle By Name(cluster=T4 {"name"="", "Variant"=variant} ("message"), "name"="shut_down") -> (w333:T4)
        n135 = Enqueue Element At Opposite End(queue=w329, element=w333) -> ()  [unwired: 2 in, 3 out]
        n136 = call <instrlib>:"Reset.vi"("error in (no error)"=w322, "VISA resource name"=w321) -> ("error out"=w319:errorcluster, "VISA resource name out"=w320:refnum<visa-resource-name>)  [unwired: 8 in]
        n137 = call <instrlib>:"Close.vi"("error in (no error)"=w319, "VISA resource name"=w320) -> ("error out"=w325:errorcluster)  [unwired: 9 in]
        n138 = Merge Errors(w325, w326) -> (w324:errorcluster)
        n139 = Bundle By Name(cluster=w328, "error in"=w324) -> (w327:T3)
      }
      frame "shut_down" {
        w339 = waveform(dbl)[] [] ("History Data")
        w344 = 0.0
        n140 = Unbundle By Name(w343) -> ("error in"=w342:errorcluster)
        n141 = property on="output 1" class="WFChart (strict)"("History Data"=w339) -> ()  [unwired: 2 in, 2 out]
        n142 = property on="output view" class="WFChart (strict)"("History Data"=w339) -> ()  [unwired: 2 in, 2 out]
        n143 = property on="output 2" class="WFChart (strict)"("History Data"=w339) -> ()  [unwired: 2 in, 2 out]
        n144 = property on="signal and timing" class="WFChart (strict)"("History Data"=waveform(dbl)[][] []) -> ()  [unwired: 2 in, 2 out]
        n145 = call <vilib>:"Simple Error Handler.vi"("error in (no error)"=w342) -> ()  [unwired: 4 in, 5 out]
        n146 = local write "Q2"(w344) -> ()
        n147 = local write "Q1"(w344) -> ()
        n148 = local write "V1"(w344) -> ()
        n149 = local write "V2"(w344) -> ()
        n150 = local write "dQ2"(w344) -> ()
        n151 = local write "dV2"(w344) -> ()
        n152 = local write "dQ1"(w344) -> ()
        n153 = local write "dV1"(w344) -> ()
      }
    }
  }
  n154 = Release Queue(queue=w3) -> ()  [unwired: 2 in, 3 out]
  n155 = property on="Status" class="Str"("Value"=w1) -> ()  [unwired: 2 in, 2 out]
